vi "top地址搜索（读取xsl）.vi"() -> ()   [LabVIEW 2020]
uses:
  1638d9b2-eac1-4fca-95b9-b72633f13618.vi
  0e5b25e2-304a-4657-9c1e-3c6bcfb22b21.vi
  d854b5f1-db06-454c-9a42-fd7535922a4b.vi
  <vilib>/Utility/file.llb/Read Delimited Spreadsheet (string).vi
  <vilib>/Comparison/Equal/Equal Functor/Equal Functor.lvclass
panel:
  out "大小":i32
  in  "eth路径 2":path=path "D:/NI 资源包/2-币猎人-事件状态机930/source/网址私钥获取/btc搜寻器/top 账号数据"
  in  "btc路径 3":path=path "D:/NI 资源包/2-币猎人-事件状态机930/source/网址私钥获取/btc搜寻器/top btc 账号数据"
  out "eth":string
  out "btc2":string
  out "btc1":string
  out "all rows 3":string[][](array[string]) caption="所有行"
  out "数组 2":string[][](array[string])
  out "index of element 2":i32 caption="元素索引"
  in  "file path (dialog if empty) 2":path=path "D:/NI 资源包/2-币猎人-事件状态机930/source/网址私钥获取/btc搜寻器/规则秘钥器/规则秘钥质数400-450.txt" caption="文件路径 （空时为对话框）"
  in  "停止":bool
  out "数组":string[][](array[string])
  out "数值 2":i32
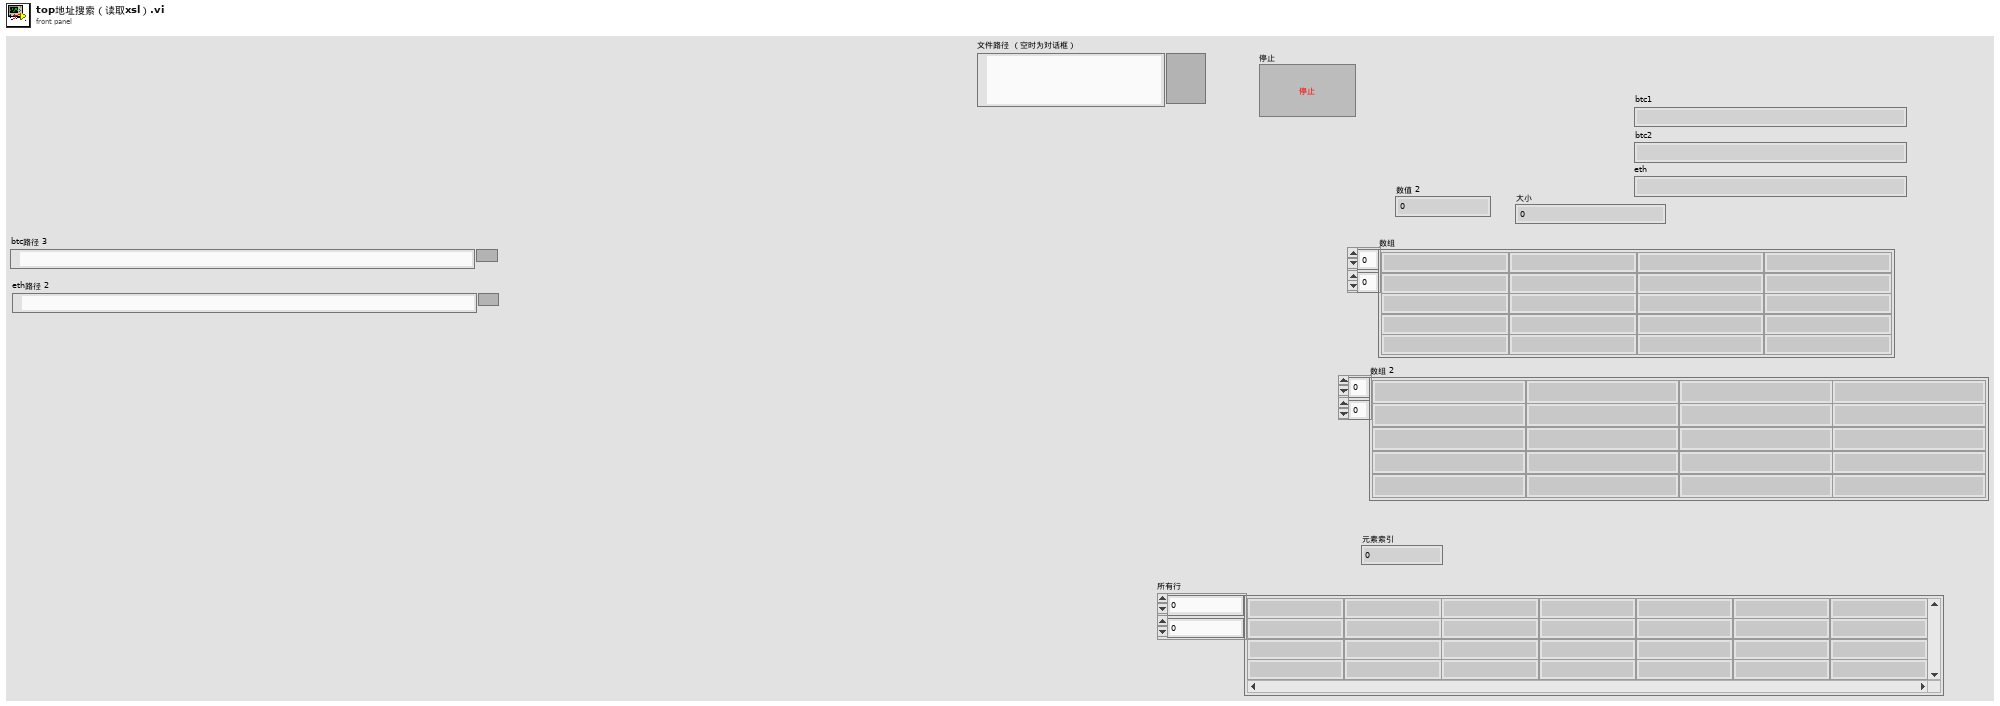
[diagram p1: front panel]
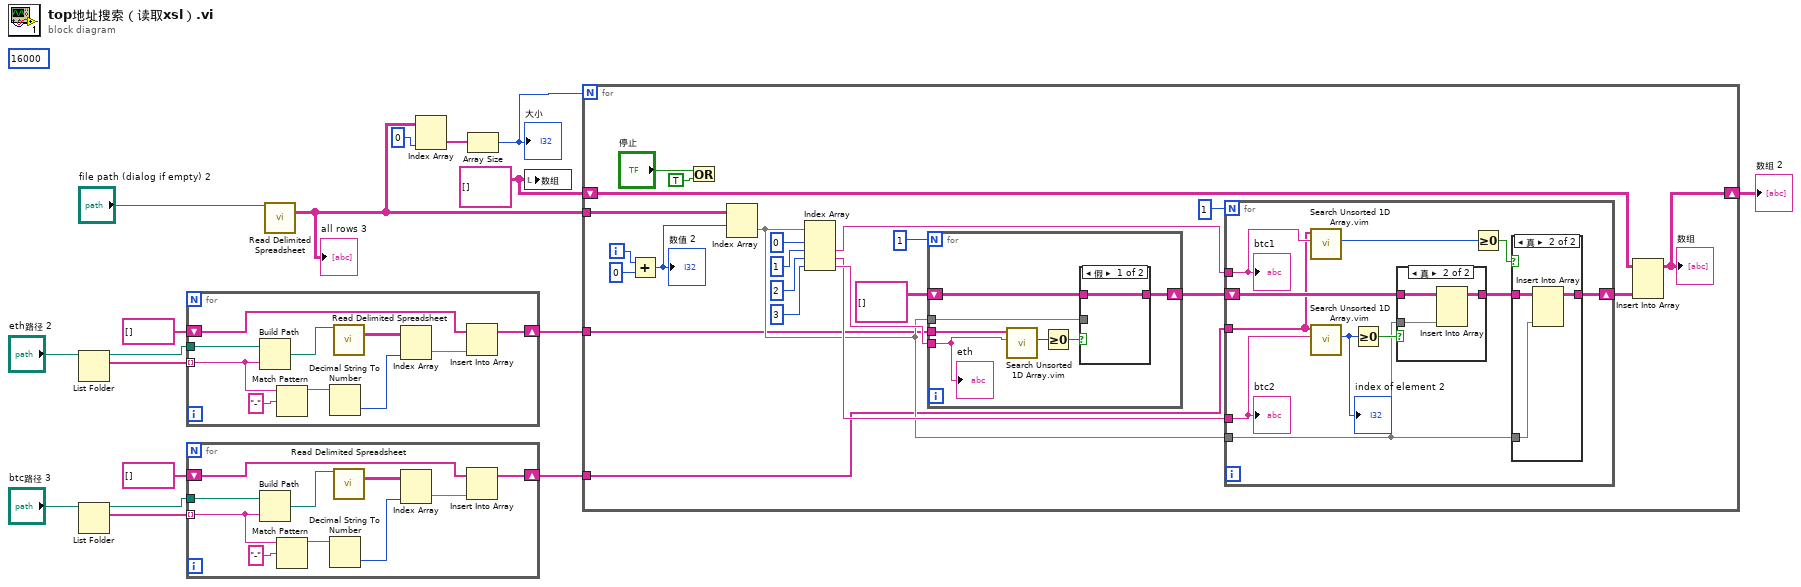
[diagram p0: block diagram]
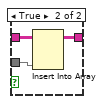
[diagram p4: hidden frame]
diagram:
  (unwired) 16000
  w17 = string[][] []
  n1 = List Folder(path="eth路径 2") -> (path out=w8:path, filenames=w9:string[])  [unwired: 3 in, 2 out]
  n2 = List Folder(path="btc路径 3") -> (path out=w13:path, filenames=w14:string[])  [unwired: 3 in, 2 out]
  n3 = for {
    tunnel: w9 -> [w22] mode=indexing
    tunnel: w8 -> [w27]
    shift-right: [w18] -> w6
    shift-left: string[] [] -> [w19]
    n4 = Build Path(base path=w27, name or relative path=w22) -> (appended path=w26:path)
    n5 = Match Pattern(string=w22, regular expression="-" ("正则表达式")) -> (before substring=w24:string)  [unwired: 1 in, 3 out]
    n6 = Decimal String To Number(string=w24) -> (number=w21:i32)  [unwired: 2 in, 1 out]
    n7 = call-poly <vilib>:"Read Delimited Spreadsheet.vi"("file path (dialog if empty)"=w26) -> ("all rows"=w25:string[][])  [unwired: 9 in, 5 out]
    n8 = Index Array(array=w25, index (col)=w21) -> (element=w20:string[])  [unwired: 1 in]
    n9 = Insert Into Array(array=w19, new element=w20) -> (w18:string[])  [unwired: 1 in]
  }
  n10 = for {
    tunnel: w14 -> [w32] mode=indexing
    tunnel: w13 -> [w37]
    shift-right: [w28] -> w11
    shift-left: string[] [] -> [w29]
    n11 = Build Path(base path=w37, name or relative path=w32) -> (appended path=w36:path)
    n12 = Match Pattern(string=w32, regular expression="-" ("正则表达式")) -> (before substring=w34:string)  [unwired: 1 in, 3 out]
    n13 = Decimal String To Number(string=w34) -> (number=w31:i32)  [unwired: 2 in, 1 out]
    n14 = call-poly <vilib>:"Read Delimited Spreadsheet.vi"("file path (dialog if empty)"=w36) -> ("all rows"=w35:string[][])  [unwired: 9 in, 5 out]
    n15 = Index Array(array=w35, index (col)=w31) -> (element=w30:string[])  [unwired: 1 in]
    n16 = Insert Into Array(array=w29, new element=w30) -> (w28:string[])  [unwired: 1 in]
  }
  n17 = call-poly <vilib>:"Read Delimited Spreadsheet.vi"("file path (dialog if empty)"="file path (dialog if empty) 2") -> ("all rows"=w4:string[][])  [unwired: 9 in, 5 out]
  "all rows 3" <- w4
  n18 = Index Array(array=w4, index (col)=0 ("禁用的索引 (列)")) -> (element=w2:string[])  [unwired: 1 in]
  n19 = Array Size(array=w2) -> (size(s)=w1:i32)
  "大小" <- w1
  n20 = local write "数组"(w17) -> ()
  n21 = for {
    N: w1 -> [_]
    shift-right: [w43] -> w16
    shift-left: w17 -> [w59]
    tunnel: w4 -> [w55]
    tunnel: w11 -> [w41]
    tunnel: w6 -> [w39]
    i -> [w46]
    n22 = Add(x=w46, y=0) -> (x+y=w42:i32)
    "数值 2" <- w42
    n23 = Or(x="停止", y=TRUE) -> ()  [unwired: 1 out]
    n24 = Index Array(array=w55, index (row)=w42) -> (element=w47:string[])  [unwired: 1 in]
    n25 = Index Array(array=w47, index #1=0 ("禁用的索引 (列)"), index #2=1 ("禁用的索引 (列)"), index #3=2 ("禁用的索引 (列)"), index #4=3 ("禁用的索引 (列)")) -> (element #2=w49:string, element #3=w48:string, element #4=w50:string)  [unwired: 1 out]
    n26 = for {
      N: 1 -> [_]
      shift-right: [w84] -> w45
      shift-left: string[][] [] -> [w86]
      tunnel: w50 -> [w83]
      tunnel: w47 -> [w81]
      tunnel: w39 -> [w80]
      n27 = call "Search Unsorted 1D Array.vim"("element"=w83, "unsorted 1D array"=w80) -> ("index of element"=w85:i32)  [unwired: 9 in]
      n28 = Greater Or Equal To 0?(x=w85) -> (x >= 0?=w82:bool)
      n29 = case shown="假" w82 {
        tunnel: w86 -> [w87 w90]
        tunnel: [w87 w89] -> w84
        tunnel: w81 -> [_ w88]
        frame False {
        }
        frame True {
          n30 = Insert Into Array(array=w90, new element=w88) -> (w89:string[][])  [unwired: 2 in]
        }
      }
      "eth" <- w83
    }
    n31 = for {
      N: 1 -> [_]
      shift-right: [w69] -> w44
      shift-left: w45 -> [w71]
      tunnel: w48 -> [w62]
      tunnel: w49 -> [w63]
      tunnel: w47 -> [w64]
      tunnel: w41 -> [w61]
      n32 = call "Search Unsorted 1D Array.vim"("element"=w63, "unsorted 1D array"=w61) -> ("index of element"=w67:i32)  [unwired: 9 in]
      n33 = call "Search Unsorted 1D Array.vim"("element"=w62, "unsorted 1D array"=w61) -> ("index of element"=w68:i32)  [unwired: 9 in]
      "index of element 2" <- w68
      n34 = Greater Or Equal To 0?(x=w68) -> (x >= 0?=w65:bool)
      n35 = case shown="真" w65 {
        tunnel: w71 -> [w76 w79]
        tunnel: [w76 w78] -> w70
        tunnel: w64 -> [_ w77]
        frame False {
        }
        frame True {
          n36 = Insert Into Array(array=w79, new element=w77) -> (w78:string[][])  [unwired: 2 in]
        }
      }
      n37 = Greater Or Equal To 0?(x=w67) -> (x >= 0?=w66:bool)
      n38 = case shown="真" w66 {
        tunnel: w70 -> [w72 w75]
        tunnel: [w72 w74] -> w69
        tunnel: w64 -> [_ w73]
        frame False {
        }
        frame True {
          n39 = Insert Into Array(array=w75, new element=w73) -> (w74:string[][])  [unwired: 2 in]
        }
      }
      "btc1" <- w63
      "btc2" <- w62
    }
    n40 = Insert Into Array(array=w59, new element=w44) -> (w43:string[][])  [unwired: 2 in]
    "数组" <- w43
  }
  "数组 2" <- w16
